vi "LEBITVacuum.InitializeSet.vi"(0 "i ref in":refnum<vi>, 2 "i attribute in":T4={"setValuePLC"=[], "nickNames"=[], "setValuePLCServiceID"=[], "monValuePLC"=[], "SetValueServiceID"=[], "MonValueServiceID"=[], "SetValue"=[], "AllPLCValues"=[], "CondSpecial2DArray"=[], "CondSpecialIndex"=[], "ReasonForLocking"="", "ReasonForLockingID"=0, "enableValuePLC"=[], "OverwriteCloseSafetyPLC"=[], "OverwriteOpenSafetyPLC"=[], "OverwriteCloseSafetyPLCServiceID"=[], "OverwriteOpenSafetyPLCServiceID"=[], "MKS Address Array"=[], "MKS MeasurementServiceID"=[], "MKS Measurement"=[], "CRYO Measurement"=[], "CRYO MeasurementServiceID"=[], "Special"=[], "Start Date"="", "MKS VISA resource"="COM13", "CRYO VISA resource"="COM13"}, 5 "error in":errorcluster) -> (14 "i ref out":refnum<vi>, 16 "i attribute out":T4={"setValuePLC"=[], "nickNames"=[], "setValuePLCServiceID"=[], "monValuePLC"=[], "SetValueServiceID"=[], "MonValueServiceID"=[], "SetValue"=[], "AllPLCValues"=[], "CondSpecial2DArray"=[], "CondSpecialIndex"=[], "ReasonForLocking"="", "ReasonForLockingID"=0, "enableValuePLC"=[], "OverwriteCloseSafetyPLC"=[], "OverwriteOpenSafetyPLC"=[], "OverwriteCloseSafetyPLCServiceID"=[], "OverwriteOpenSafetyPLCServiceID"=[], "MKS Address Array"=[], "MKS MeasurementServiceID"=[], "MKS Measurement"=[], "CRYO Measurement"=[], "CRYO MeasurementServiceID"=[], "Special"=[], "Start Date"="", "MKS VISA resource"="COM13", "CRYO VISA resource"="COM13"}, 19 "error out":errorcluster)   [LabVIEW 2014, in "LEBITVacuum.lvlib"]
uses:
  LEBITVacuum.lvlib
  CS_Core/CSSystem/CoreDefs/CoreDefs.call_type.ctl
  CS_Core/BaseProcess/BaseProcess.descriptor string definition.ctl
  CS_Core/CSSystem/CoreDefs/CoreDefs.rawDataType.ctl
  LEBITVacuum.i attribute.ctl
  CSlibraries/UtilityLib/UtilityLib.valueStatus.ctl
  CS_Core/CSSystem/CoreLib/CoreLib.string 2 byte array.vi
  CS_Core/CSSystem/CoreLib/CoreLib.byte array 2 short.vi
  CSlibraries-extern/DimLVEvent/LVDimInterface/LVDimInterface.lvlib
  CS_Core/CSSystem/CoreLib/CoreLib.lvlib
  CSlibraries/UtilityLib/UtilityLib.lvlib
  CS_Core/BaseProcess/BaseProcess.lvlib
panel:
  in  "call cluster in":T1={"Object"="", "Selector"="", "CallType"=enum."synchronous", "Async Object"="", "Async Selector"="", "Data Descriptor"="", "Data"=[], "Error #"=0, "Expire"=0}
  out "setValuePLC":string
  out "SetValue":i16
  in  "call cluster in":T1={"Object"="", "Selector"="", "CallType"=enum."synchronous", "Async Object"="", "Async Selector"="", "Data Descriptor"="", "Data"=[], "Error #"=0, "Expire"=0}
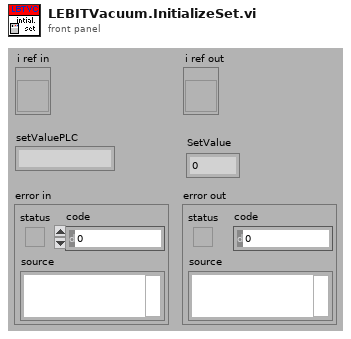
[diagram p1: front panel]
types:
  T1 = typedef "CoreDefs.call_type.ctl" = cluster{"Object":string, "Selector":string, "CallType":enum16{"simple", "synchronous", "asynchronous"}, "Async Object":string, "Async Selector":string, "Data Descriptor":T2, "Data":T3, "Error #":i32, "Expire":u32}
  T2 = typedef "BaseProcess.lvlib/BaseProcess.descriptor string definition.ctl" = string
  T3 = typedef "CoreDefs.rawDataType.ctl" = i8[]
  T4 = typedef "LEBITVacuum.lvlib/LEBITVacuum.i attribute.ctl" = cluster{"setValuePLC":string[], "nickNames":string[], "setValuePLCServiceID":i32[], "monValuePLC":string[], "SetValueServiceID":i32[], "MonValueServiceID":i32[], "SetValue":i16[], "AllPLCValues":string[], "CondSpecial2DArray":string[][], "CondSpecialIndex":i32[], "ReasonForLocking":string, "ReasonForLockingID":i32, "enableValuePLC":string[], "OverwriteCloseSafetyPLC":string[], "OverwriteOpenSafetyPLC":string[], "OverwriteCloseSafetyPLCServiceID":i32[], "OverwriteOpenSafetyPLCServiceID":i32[], "MKS Address Array":i32[][], "MKS MeasurementServiceID":i32[], "MKS Measurement":string[], "CRYO Measurement":string[][], "CRYO MeasurementServiceID":i32[], "Special":string[], "Start Date":string, "MKS VISA resource":refnum<visa-resource-name>, "CRYO VISA resource":refnum<visa-resource-name>}
  T5 = typedef "UtilityLib.lvlib/UtilityLib.valueStatus.ctl" = enum16{"no info available", "stand by/off", "on", "warning", "alarm/malfunction", "not implemented", "user action required", "important information", "system default", "control default", "indicator default", "button default"}
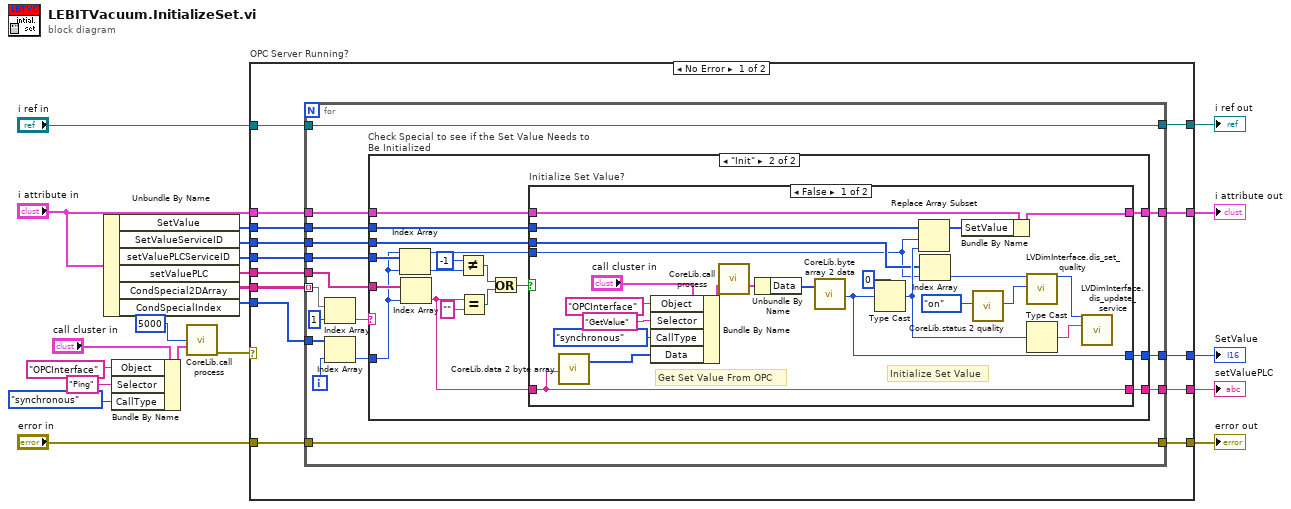
[diagram p0: block diagram]
diagram:
  n1 = Unbundle By Name("i attribute in") -> ("SetValue"=w19:i16[], "SetValueServiceID"=w18:i32[], "setValuePLCServiceID"=w17:i32[], "setValuePLC"=w21:string[], "CondSpecial2DArray"=w16:string[][], "CondSpecialIndex"=w15:i32[])
  n2 = Bundle By Name(cluster="call cluster in", "Object"="OPCInterface", "Selector"="Ping" ("string"), "CallType"=enum16{"simple", "synchronous", "asynchronous"}."synchronous") -> (w9:T1)
  n3 = call "CoreLib.call process.vi"("timeout (ms)"=5000, "call cluster in"=w9) -> ("error out"=w6:errorcluster)  [unwired: 12 in, 1 out]
  n4 = case "OPC Server Running?" shown="No Error" w6 {
    tunnel: w21 -> [w35 _]
    tunnel: "i attribute in" -> [w34 w95]
    tunnel: w19 -> [w33 _]
    tunnel: w18 -> [w32 _]
    tunnel: w17 -> [w31 _]
    tunnel: w16 -> [w30 _]
    tunnel: w15 -> [w29 _]
    tunnel: "i ref in" -> [w28 w96]
    tunnel: "error in" -> [w27 w94]
    tunnel: [w26 w96] -> w5
    tunnel: [w25 w95] -> w4
    tunnel: [w24 _] -> w3
    tunnel: [w23 _] -> w2
    tunnel: [w22 w94] -> w1
    frame No Error {
      n5 = for {
        tunnel: w35 -> [w51]
        tunnel: [w50] -> w25
        tunnel: w34 -> [w49]
        tunnel: w33 -> [w48]
        tunnel: w32 -> [w47]
        tunnel: w31 -> [w46]
        tunnel: [w45] -> w23
        tunnel: [w44] -> w24
        tunnel: w30 -> [w42] mode=indexing
        tunnel: w29 -> [w39]
        tunnel: w28 -> [w37]
        tunnel: [w37] -> w26
        tunnel: w27 -> [w36]
        tunnel: [w36] -> w22
        i -> [w38]
        n6 = Index Array(array=w42, index=1) -> (element=w43:string)
        n7 = Index Array(array=w39, index=w38) -> (element=w40:i32)
        n8 = case "Check Special to see if the Set Value Needs to Be Initialized" shown="\"Init\"" w43 {
          tunnel: w51 -> [_ w66]
          tunnel: [w52 w62] -> w50
          tunnel: w49 -> [w52 w61]
          tunnel: w48 -> [_ w60]
          tunnel: w47 -> [_ w59]
          tunnel: w46 -> [_ w57]
          tunnel: [_ w55] -> w45
          tunnel: [_ w54] -> w44
          tunnel: w40 -> [_ w53]
          frame "", Default {
          }
          frame "Init" {
            n9 = Index Array(array=w57, index=w53) -> (element=w65:i32)
            n10 = Index Array(array=w66, index=w53) -> (element=w56:string)
            n11 = Not Equal?(x=-1 ("y"), y=w65) -> (x != y?=w64:bool)
            n12 = Equal?(x=w56, y="") -> (x = y?=w68:bool)
            n13 = Or(x=w64, y=w68) -> (x .or. y?=w63:bool)
            n14 = case "Initialize Set Value?" shown="False" w63 {
              tunnel: w59 -> [w84 _]
              tunnel: w60 -> [w85 _]
              tunnel: w53 -> [w83 _]
              tunnel: w61 -> [w91 w93]
              tunnel: [w88 w93] -> w62
              tunnel: w56 -> [w74 w92]
              tunnel: [w74 w92] -> w55
              tunnel: [w73 _] -> w54
              frame False {
                # "Initialize Set Value"
                # "Get Set Value From OPC"
                n15 = call-poly "CoreLib.data 2 byte array.vi"("string"=w74) -> ("byteArray out"=w79:T3)  [unwired: 18 in]
                n16 = Bundle By Name(cluster="call cluster in", "Object"="OPCInterface", "Selector"="GetValue" ("string"), "CallType"=enum16{"simple", "synchronous", "asynchronous"}."synchronous", "Data"=w79) -> (w82:T1)
                n17 = call "CoreLib.call process.vi"("call cluster in"=w82) -> ("call cluster out"=w76:T1)  [unwired: 13 in, 1 out]
                n18 = Unbundle By Name(w76) -> ("Data"=w75:T3)
                n19 = call-poly "CoreLib.byte array 2 data.vi"("byteArray"=w75) -> ("i16"=w73:i16)  [unwired: 16 in, 2 out]
                n20 = Type Cast(type=i16 0, x=w73) -> (*(type *) &x=w87:i16)
                n21 = Replace Array Subset(array=w85, new element=w87, index=w83) -> (w89:i16[])
                n22 = Index Array(array=w84, index=w83) -> (element=w71:i32)
                n23 = Bundle By Name(cluster=w91, "SetValue"=w89) -> (w88:T4)
                n24 = call "CoreLib.status 2 quality.vi"("valueStatus"=UtilityLib.valueStatus."on") -> ("quality"=w72:i32)  [unwired: 18 in]
                n25 = call "LVDimInterface.dis_set_quality.vi"("my_serviceID"=w71, "quality"=w72) -> ("my_serviceID (out)"=w69:i32)  [unwired: 16 in, 1 out]
                n26 = Type Cast(x=w87) -> (*(type *) &x=w86:string)  [unwired: 1 in]
                n27 = call "LVDimInterface.dis_update_service.vi"("my_serviceID"=w69, "data"=w86) -> ()  [unwired: 15 in, 3 out]
              }
              frame True {
              }
            }
          }
        }
      }
    }
    frame Error {
      # "OPC Server Not Running!"
    }
  }
  "i attribute out" <- w4
  "setValuePLC" <- w2
  "SetValue" <- w3
  "i ref out" <- w5
  "error out" <- w1
